vi "Implement Publication Policy.vi"(5 "Last Published Value":variant, 7 "Last Published Time":timestamp, 9 "New Value Time":timestamp, 10 "New Value":variant, 11 "PublicationPolicy":refnum<class "IPublicationPolicy.lvclass">) -> (0 "error out (Reject Publication)":errorcluster, 2 "Value to Publish":variant)   [LabVIEW 2017, in "IMediator.lvlib" / "IPublicationPolicy.lvclass"]
doc: "This method decides whether or not to send or otherwise handle the new data value. The policy is set and maintained by the subscriber. The Topic Actor knows no policy details, it just passes the new value in. If there is a failure inside this method, the Topic Actor must assume the listener is no longer valid (dead/unrecoverable) and should delete it from the Subscriber list.\n\n<License>\nCopyright © 2017 Composed Systems, LLC | All rights reserved\nwww.composed.io\n\nAuthor: Ethan Stern <ethan.stern@composed.io>\n\nThis software is provided \"AS IS\" WITHOUT WARRANTIES, either express or implied, AND IS FOR EDUCATIONAL PURPOSES ONLY.\n</License>"
uses:
  IPublicationPolicy.lvclass
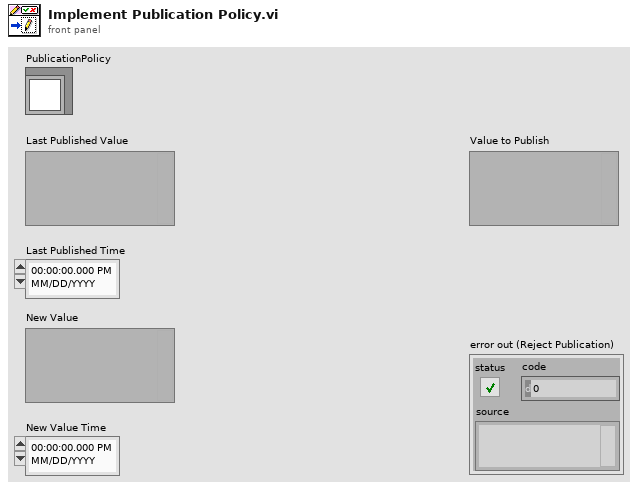
[diagram p1: front panel]
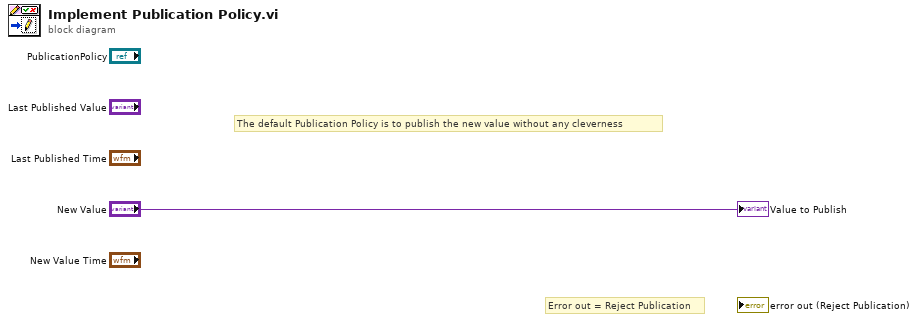
[diagram p0: block diagram]
diagram:
  # "The default Publication Policy is to publish the new value without any cleverness"
  # "Error out = Reject Publication"
  "Value to Publish" <- "New Value"
